vi "PH_Switch.calc PSDB Status Data.vi"(0 "Status":T1 items=["no info", "off/false/out", "on/true/in", "Failure", "Alarm", "Status 1", "Status 2", "Status 3"], 5 "caption false":string, 7 "caption true":string, 9 "Tagname false":string, 11 "Tagname true":string) -> (8 "PSDB Status":string)   [LabVIEW 2014, in "PH_Switch.lvlib"]
uses:
  PH_Switch.lvlib
  PH_Basics/PH_StatusHandler/PH_StatusHandler.Status.ctl
  PH_Basics/PH_StatusHandler/PH_StatusHandler.lvlib
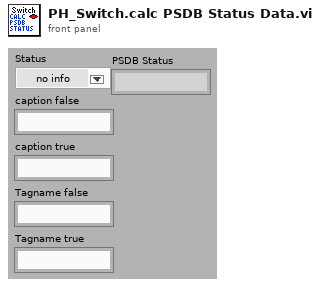
[diagram p1: front panel]
types:
  T1 = typedef "PH_StatusHandler.lvlib/PH_StatusHandler.Status.ctl" = i16
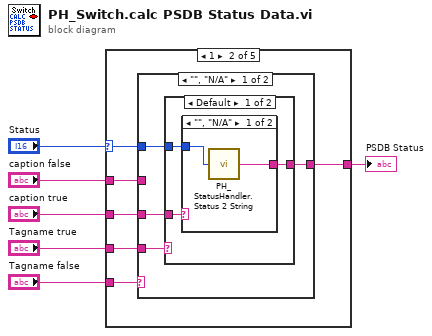
[diagram p0: block diagram]
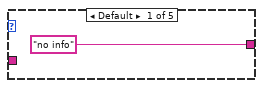
[diagram p2: hidden frame]
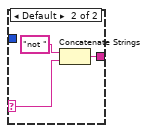
[diagram p3: hidden frame]
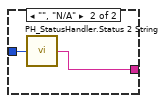
[diagram p4: hidden frame]
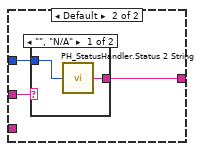
[diagram p5: hidden frame]
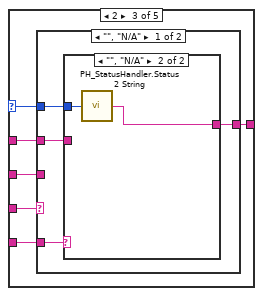
[diagram p7: hidden frame]
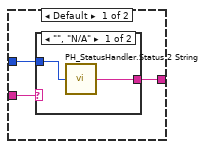
[diagram p8: hidden frame]
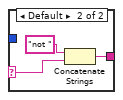
[diagram p9: hidden frame]
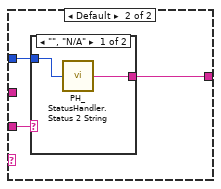
[diagram p10: hidden frame]
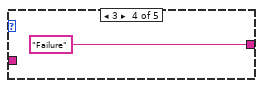
[diagram p12: hidden frame]
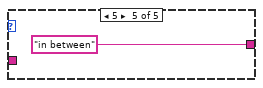
[diagram p13: hidden frame]
diagram:
  n1 = case shown="1" "Status" {
    selector: "Status" -> [_ w8 w38 _ _]
    tunnel: "caption false" -> [_ w11 w35 _ _]
    tunnel: "caption true" -> [_ w9 w36 _ _]
    tunnel: ["no info" ("Caption In") w12 w39 "Failure" ("Caption In") "in between" ("Caption In")] -> w4
    tunnel: "Tagname true" -> [_ w10 w37 _ _]
    tunnel: "Tagname false" -> [_ w13 w34 _ _]
    frame Default {
    }
    frame 1 {
      n2 = case shown="\"\", \"N/A\"" w13 {
        tunnel: [w15 w29] -> w12
        tunnel: w11 -> [_ w30]
        tunnel: w10 -> [w17 _]
        tunnel: w9 -> [w16 _]
        tunnel: w8 -> [w14 w28]
        frame "", "N/A" {
          n3 = case shown="Default" w17 {
            tunnel: w16 -> [w19 _]
            tunnel: [w20 w26] -> w15
            tunnel: w14 -> [w18 w27]
            frame Default {
              n4 = case shown="\"\", \"N/A\"" w19 {
                selector: w19 -> [_ w23]
                tunnel: [w21 w24] -> w20
                tunnel: w18 -> [w22 _]
                frame "", "N/A" {
                  n5 = call "PH_StatusHandler.Status 2 String.vi"("Status"=w22) -> ("Status as string"=w21:string)
                }
                frame Default {
                  n6 = Concatenate Strings("not " ("string"), w23) -> (w24:string)
                }
              }
            }
            frame "", "N/A" {
              n7 = call "PH_StatusHandler.Status 2 String.vi"("Status"=w27) -> ("Status as string"=w26:string)
            }
          }
        }
        frame Default {
          n8 = case shown="\"\", \"N/A\"" w30 {
            selector: w30 -> [_ w33]
            tunnel: [w31 w33] -> w29
            tunnel: w28 -> [w32 _]
            frame "", "N/A" {
              n9 = call "PH_StatusHandler.Status 2 String.vi"("Status"=w32) -> ("Status as string"=w31:string)
            }
            frame Default {
            }
          }
        }
      }
    }
    frame 2 {
      n10 = case shown="\"\", \"N/A\"" w37 {
        tunnel: [w41 w55] -> w39
        tunnel: w36 -> [_ w56]
        tunnel: w34 -> [w43 _]
        tunnel: w35 -> [w42 _]
        tunnel: w38 -> [w40 w54]
        frame "", "N/A" {
          n11 = case shown="\"\", \"N/A\"" w43 {
            tunnel: w42 -> [w45 _]
            tunnel: [w46 w52] -> w41
            tunnel: w40 -> [w44 w53]
            frame Default {
              n12 = case shown="\"\", \"N/A\"" w45 {
                selector: w45 -> [_ w49]
                tunnel: [w47 w50] -> w46
                tunnel: w44 -> [w48 _]
                frame "", "N/A" {
                  n13 = call "PH_StatusHandler.Status 2 String.vi"("Status"=w48) -> ("Status as string"=w47:string)
                }
                frame Default {
                  n14 = Concatenate Strings("not " ("string"), w49) -> (w50:string)
                }
              }
            }
            frame "", "N/A" {
              n15 = call "PH_StatusHandler.Status 2 String.vi"("Status"=w53) -> ("Status as string"=w52:string)
            }
          }
        }
        frame Default {
          n16 = case shown="\"\", \"N/A\"" w56 {
            selector: w56 -> [_ w59]
            tunnel: [w57 w59] -> w55
            tunnel: w54 -> [w58 _]
            frame "", "N/A" {
              n17 = call "PH_StatusHandler.Status 2 String.vi"("Status"=w58) -> ("Status as string"=w57:string)
            }
            frame Default {
            }
          }
        }
      }
    }
    frame 3 {
    }
    frame 5 {
    }
  }
  "PSDB Status" <- w4
